vi "Ballard XML Generator.Add Parameter Properties.vi"(0 "signed? (T)":bool=TRUE, 1 "default value":string, 4 "offset (0)":string, 5 "units (psi)":string="psi", 6 "scale (1)":string, 7 "encoding (BNR)":T1, 8 "number of bits":i32, 9 "start bit":i32, 10 "name":string, 11 "string in":string) -> (3 "string out":string)   [LabVIEW 2017]
uses:
  Controls/Encoding.ctl
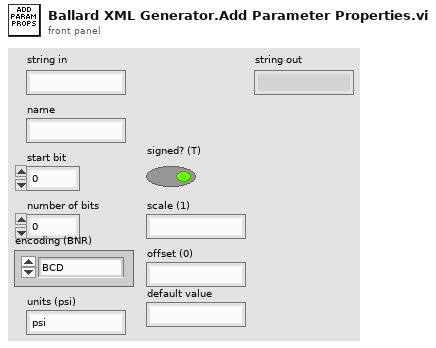
[diagram p1: front panel]
types:
  T1 = typedef "Encoding.ctl" = enum16{"BCD", "BNR", "Discrete"}
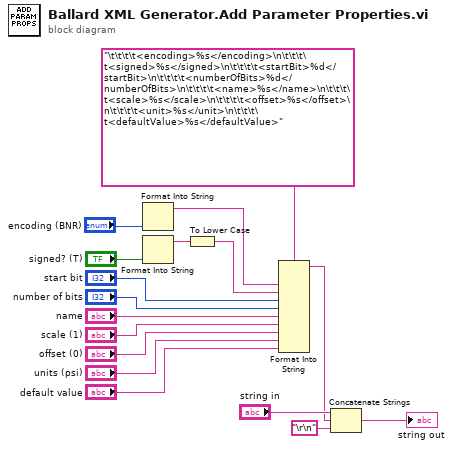
[diagram p0: block diagram]
diagram:
  n1 = Format Into String("encoding (BNR)") -> (resulting string=w3:string)  [unwired: 3 in, 1 out]
  n2 = Format Into String("signed? (T)") -> (resulting string=w11:string)  [unwired: 3 in, 1 out]
  n3 = To Lower Case(string=w11) -> (all lower case string=w4:string)
  n4 = Format Into String(format string="\t\t\t\t<encoding>%s</encoding>\n\t\t\t\t<signed>%s</signed>\n\t\t\t\t<startBit>%d</startBit>\n\t\t\t\t<numberOfBits>%d</numberOfBits>\n\t\t\t\t<name>%s</name>\n\t\t\t\t<scale>%s</scale>\n\t\t\t\t<offset>%s</offset>\n\t\t\t\t<unit>%s</unit>\n\t\t\t\t<defaultValue>%s</defaultValue>", w3, w4, "start bit", "number of bits", "name", "scale (1)", "offset (0)", "units (psi)", "default value") -> (resulting string=w13:string)  [unwired: 2 in, 1 out]
  n5 = Concatenate Strings("string in", w13, "\r\n") -> (→"string out":string)
